vi "incre-decre-botones.vi"() -> ()   [LabVIEW 2024]
panel:
  in  "stop":bool
  in  "Incremento":bool
  in  "Decremento":bool
  in  "Nada":bool
  in  "Slide":dbl(slide) scale=-3.0..3.0
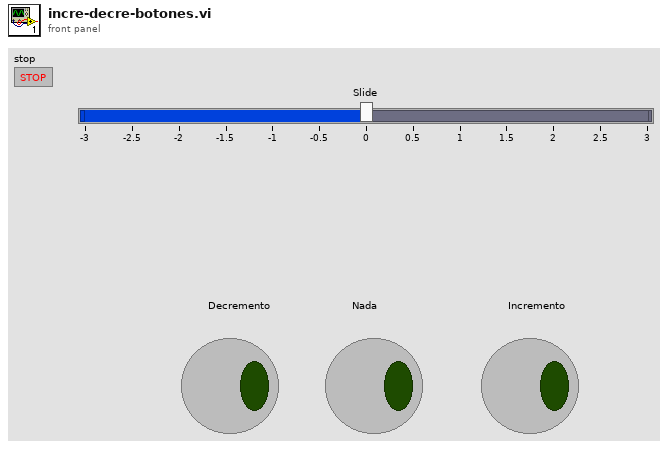
[diagram p1: front panel]
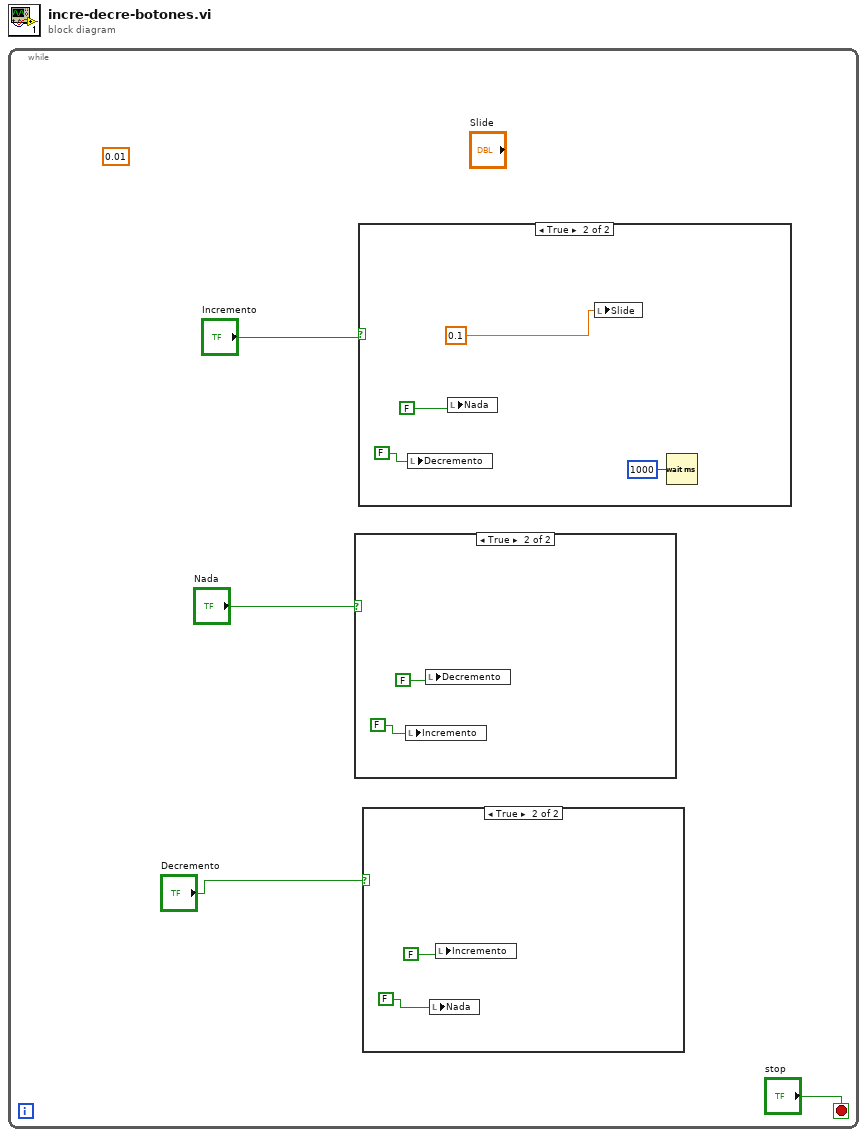
[diagram p0: block diagram]
diagram:
  n1 = while {
    stop <- "stop" stop-if-true
    (unwired) 0.01
    n2 = case shown="True" "Nada" {
      frame False {
      }
      frame True {
        n3 = local write "Incremento"(FALSE) -> ()
        n4 = local write "Decremento"(FALSE) -> ()
      }
    }
    n5 = case shown="True" "Incremento" {
      frame False {
      }
      frame True {
        n6 = local write "Decremento"(FALSE) -> ()
        n7 = local write "Nada"(FALSE) -> ()
        n8 = local write "Slide"(0.1) -> ()
        n9 = Wait (ms)(milliseconds to wait=u32 1000) -> ()  [unwired: 1 out]
      }
    }
    n10 = case shown="True" "Decremento" {
      frame False {
      }
      frame True {
        n11 = local write "Nada"(FALSE) -> ()
        n12 = local write "Incremento"(FALSE) -> ()
      }
    }
  }
